vi "Array Averager.vi"(11 "Array":dbl[](array[numeric])) -> (3 "Averaged Array":dbl)   [LabVIEW 2017]
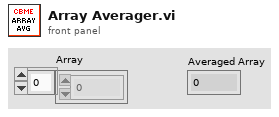
[diagram p1: front panel]
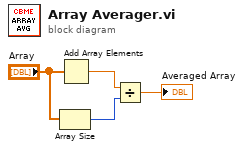
[diagram p0: block diagram]
diagram:
  n1 = Array Size(array="Array") -> (size(s)=w2:i32)
  n2 = Add Array Elements(numeric array="Array") -> (sum=w3:dbl)
  n3 = Divide(x=w3, y=w2) -> (x/y=→"Averaged Array":dbl)
